vi "Rectangular Target Robot Main.vi"() -> ()   [LabVIEW 2011]
doc: "This VI imlements the framework and scheduler for your robotics program. It should not be necessary to modify the framework. You are expected to add your code to the VIs called from Robot Main, the ones located in the Team Code within the project."
uses:
  <vilib>/Rock Robotics/WPI/Camera/WPI_CameraImageSize.ctl
  Robot Global Data.vi
panel:
  out "Target Info":T1(array[cluster])
  in  "Image Size":T2=enum."160x120"
  in  "Enable Vision":bool=TRUE
  in  "Finish":bool
  # "The button and ring selector to the left allow you to control basic camera settings.\nOnce processing is calibrated, the table below shows target position.\nOpen the block diagram for more complete instructions"
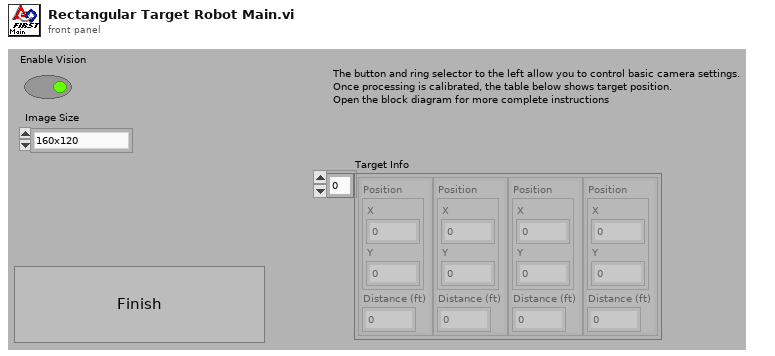
[diagram p1: front panel]
types:
  T1 = cluster{"Position":cluster{"X":dbl, "Y":dbl}, "Distance (ft)":dbl}[]
  T2 = typedef "WPI_CameraImageSize.ctl" = enum16{"640x480", "320x240", "160x120"}
  T3 = typedef "WPI_DriverStationMatch Info.ctl" = cluster{"Autonomous Elapsed Seconds":dbl, "TeleOp Elapsed Seconds":dbl, "Disabled Elapsed Seconds":dbl, "Visited Autonomous":bool, "Visited TeleOp":bool, "Visited Disabled":bool, "Autonomous Settings":cluster{"Autonomous Style":enum16{"Iterative", "Independent"}, "VI Refnum":refnum<vi>}}
  T4 = typedef "WPI_DriverStationDerivedRobotMode.ctl" = enum16{"Init", "Execute", "Stop"}
  T5 = typedef "WPI_DriverStationRobotMode.ctl" = enum16{"Autonomous Disabled", "Autonomous Enabled", "Teleop Disabled", "Teleop Enabled", "Timeout", "Finish"}
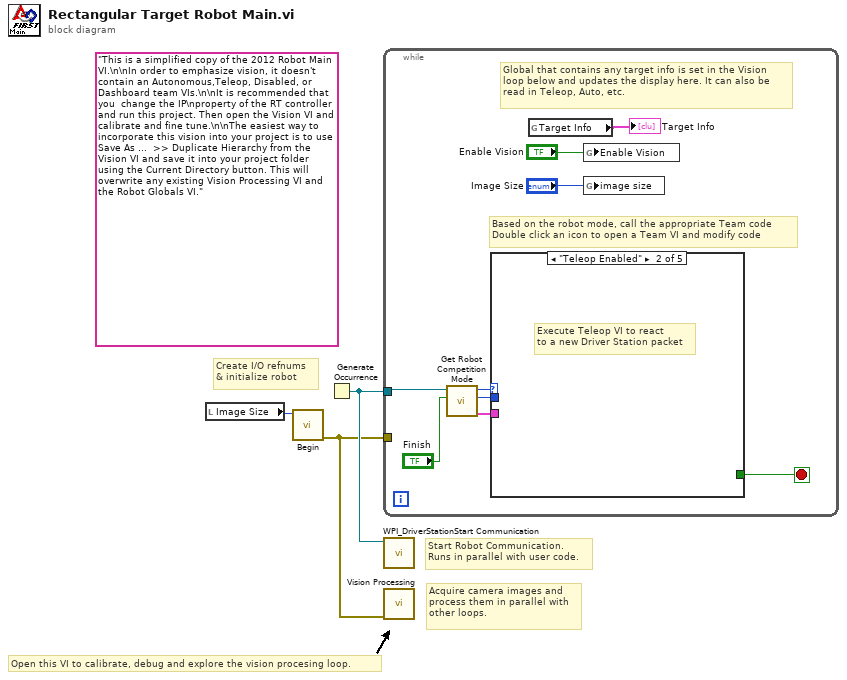
[diagram p0: block diagram]
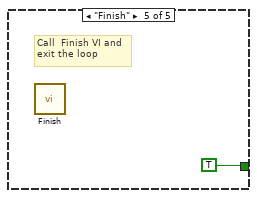
[diagram p5: hidden frame]
diagram:
  (unwired) "This is a simplified copy of the 2012 Robot Main VI.\n\nIn order to emphasize vision, it doesn't contain an Autonomous,Teleop, Disabled, or Dashboard team VIs.\n\nIt is recommended that you  change the IP\nproperty of the RT controller and run this project. Then open the Vision VI and calibrate and fine tune.\n\nThe easiest way to incorporate this vision into your project is to use Save As ...  >> Duplicate Hierarchy from the Vision VI and save it into your project folder using the Current Directory button. This will overwrite any existing Vision Processing VI and the Robot Globals VI."
  # "Open this VI to calibrate, debug and explore the vision procesing loop."
  # "Acquire camera images and\nprocess them in parallel with\nother loops."
  # "Create I/O refnums\n& initialize robot"
  # "Start Robot Communication.\nRuns in parallel with user code."
  n1 = local read "Image Size"() -> (w2:T2)
  n2 = call "Begin.vi"("Image Size"=w2) -> ("error out"=w1:errorcluster)  [unwired: 10 out]
  n3 = Generate Occurrence() -> (w3:refnum<k4>)
  n4 = while {
    tunnel: w3 -> [w10]
    tunnel: w1 -> [_]
    stop <- w7 stop-if-true
    # "Global that contains any target info is set in the Vision\nloop below and updates the display here. It can also be\nread in Teleop, Auto, etc."
    # "Based on the robot mode, call the appropriate Team code\nDouble click an icon to open a Team VI and modify code"
    n5 = call "Get Robot Competition Mode.vi"("Finish"="Finish", "DS Occurrence"=w10) -> ("Match Info out"=w8:T3, "Call Context"=w12:T4, "Robot Mode"=w11:T5)  [unwired: 7 out]
    n6 = case shown="\"Teleop Enabled\"" w11 {
      tunnel: w12 -> [_ _ _ _ _]
      tunnel: w8 -> [_ _ _ _ _]
      tunnel: [_ _ _ _ TRUE] -> w7
      frame "Autonomous Enabled" {
        # "On First Autonomous packet, start the\nAutonomous VI running in parallel.\nRemember the VI refnum.\nOn last , Stop the VI.\nNo need to respond to intermediates."
      }
      frame "Teleop Enabled" {
        # "Execute Teleop VI to react\nto a new Driver Station packet"
      }
      frame "Autonomous Disabled", "Teleop Disabled" {
        # "Execute Disabled VI in case there\nis something to  handle for a\ndisabled Driver Station packet"
      }
      frame "Timeout" {
        # "Driver Station packet didn't arrive.\nPossibly useful for diagnostics"
      }
      frame "Finish" {
        # "Call  Finish VI and\nexit the loop"
        n7 = call "Finish.vi"() -> ()  [unwired: 1 in, 7 out]
      }
    }
    n8 = global read "Robot Global Data.vi" "Target Info"() -> (→"Target Info":T1)
    n9 = global write "Robot Global Data.vi" "Enable Vision"("Enable Vision") -> ()
    n10 = global write "Robot Global Data.vi" "image size"("Image Size") -> ()
  }
  n11 = call <vilib>:"WPI_DriverStationStart Communication.vi"("occurrence"=w3) -> ()  [unwired: 11 out]
  n12 = call "Vision Processing.vi"("error in (no error)"=w1) -> ()  [unwired: 7 in]
